vi "setVIcontrolRemotelyByIndex.vi"(9 "Round to Nearest":dbl=0.5 format="%#_13g", 10 "ValueToSet":dbl, 11 "Array":cluster{"VIname":string, "controlIndex":i32}[](array[cluster])) -> ()   [LabVIEW 2021]
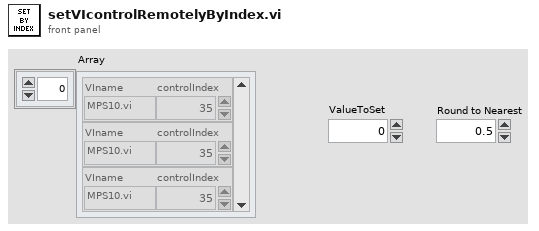
[diagram p1: front panel]
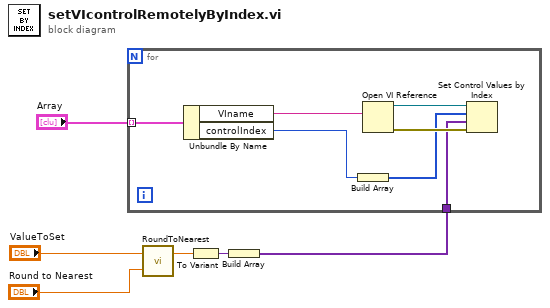
[diagram p0: block diagram]
diagram:
  n1 = call "RoundToNearest.vi"("Round to Nearest"="Round to Nearest", "Numeric"="ValueToSet") -> ("Nearest"=w3:dbl)
  n2 = To Variant(anything=w3) -> (Variant=w6:variant)
  n3 = Build Array(w6) -> (w5:variant[])
  n4 = for {
    tunnel: w5 -> [w11]
    tunnel: "Array" -> [w9] mode=indexing
    n5 = Unbundle By Name(w9) -> ("VIname"=w8:string, "controlIndex"=w7:i32)
    n6 = Build Array(w7) -> (w10:i32[])
    n7 = Open VI Reference(vi path=w8) -> (vi reference=w12:refnum<vi>, error out=w13:errorcluster)  [unwired: 5 in]
    n8 = Set Control Values by Index(0:w12, 1:w10, 2:w11, 3:w13) -> ()  [unwired: 1 out]
  }
